vi "Functions_Unload All.vi"(0 "scripts manager in":refnum<class "scripts manager.lvclass">, 11 "error in (no error)":errorcluster) -> (4 "scripts manager out":refnum<class "scripts manager.lvclass">, 15 "error out":errorcluster)   [LabVIEW 2016, in "scripts manager.lvclass"]
uses:
  scripts manager.lvclass
  common/function utils/Scan Syntax Format.ctl
  functions/functionsbase/functionbase.lvclass
  scripts manager.lvclass/scripts manager.ctl
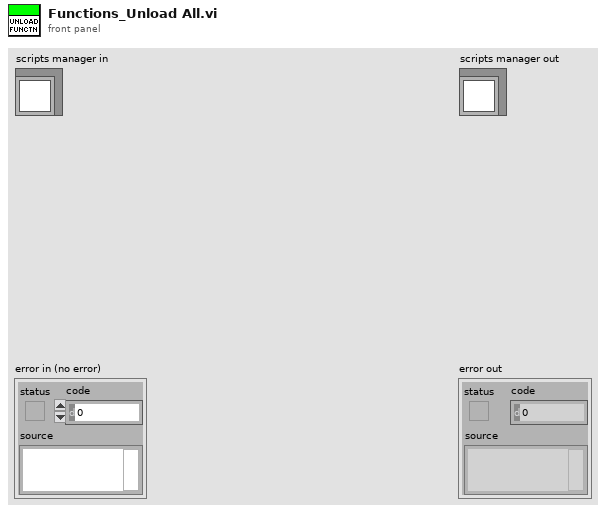
[diagram p1: front panel]
types:
  T1 = cluster{"Function Name":string[], "Function Obj":refnum<class "functionbase.lvclass">[]}
  T2 = typedef "Scan Syntax Format.ctl" = cluster{"Format String":string, "Variable#":i32, "Variables Name":string[]}
  T3 = cluster{"Function Name":string[], "Scan Syntax Format":T2[], "Smart Syntax Representation List":string[]}
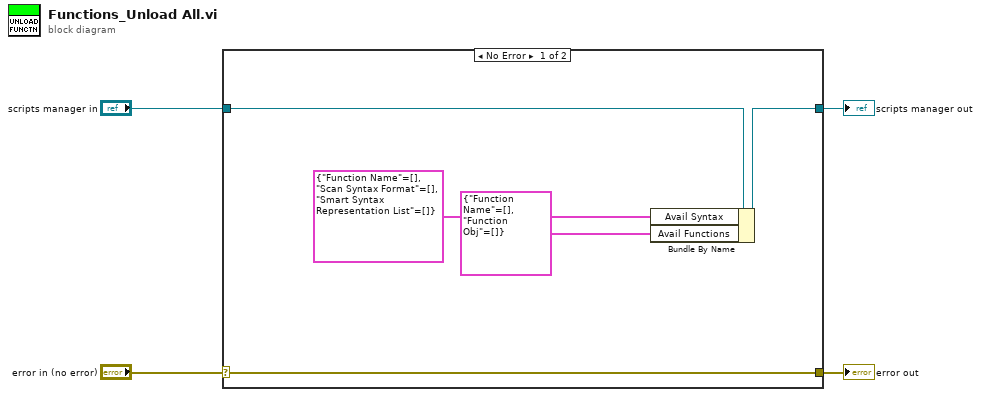
[diagram p0: block diagram]
diagram:
  n1 = case shown="No Error" "error in (no error)" {
    selector: "error in (no error)" -> [w9 w11]
    tunnel: [w9 w11] -> w3
    tunnel: [w7 w10] -> w1
    tunnel: "scripts manager in" -> [w8 w10]
    frame No Error {
      n2 = Bundle By Name(cluster=w8, "Avail Syntax"=T3 {"Function Name"=[], "Scan Syntax Format"=[], "Smart Syntax Representation List"=[]}, "Avail Functions"=T1 {"Function Name"=[], "Function Obj"=[]}) -> (w7:refnum<class "scripts manager.lvclass">)
    }
    frame Error {
    }
  }
  "error out" <- w3
  "scripts manager out" <- w1
